vi "模拟量输入自动测试一组_fast_OK.vi"(8 "AD选择？":bool, 9 "DSP选择？":bool, 11 "第几个":i32) -> ()   [LabVIEW 2010]
panel:
  in  "AD测试值":dbl[](array[numeric])
  in  "DSP测试值":dbl[](array[numeric])
  # "从0开始"
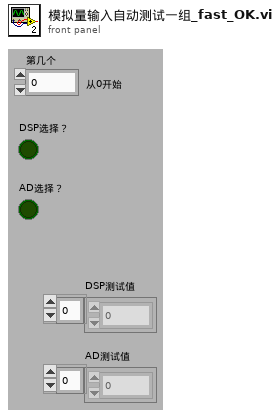
[diagram p1: front panel]
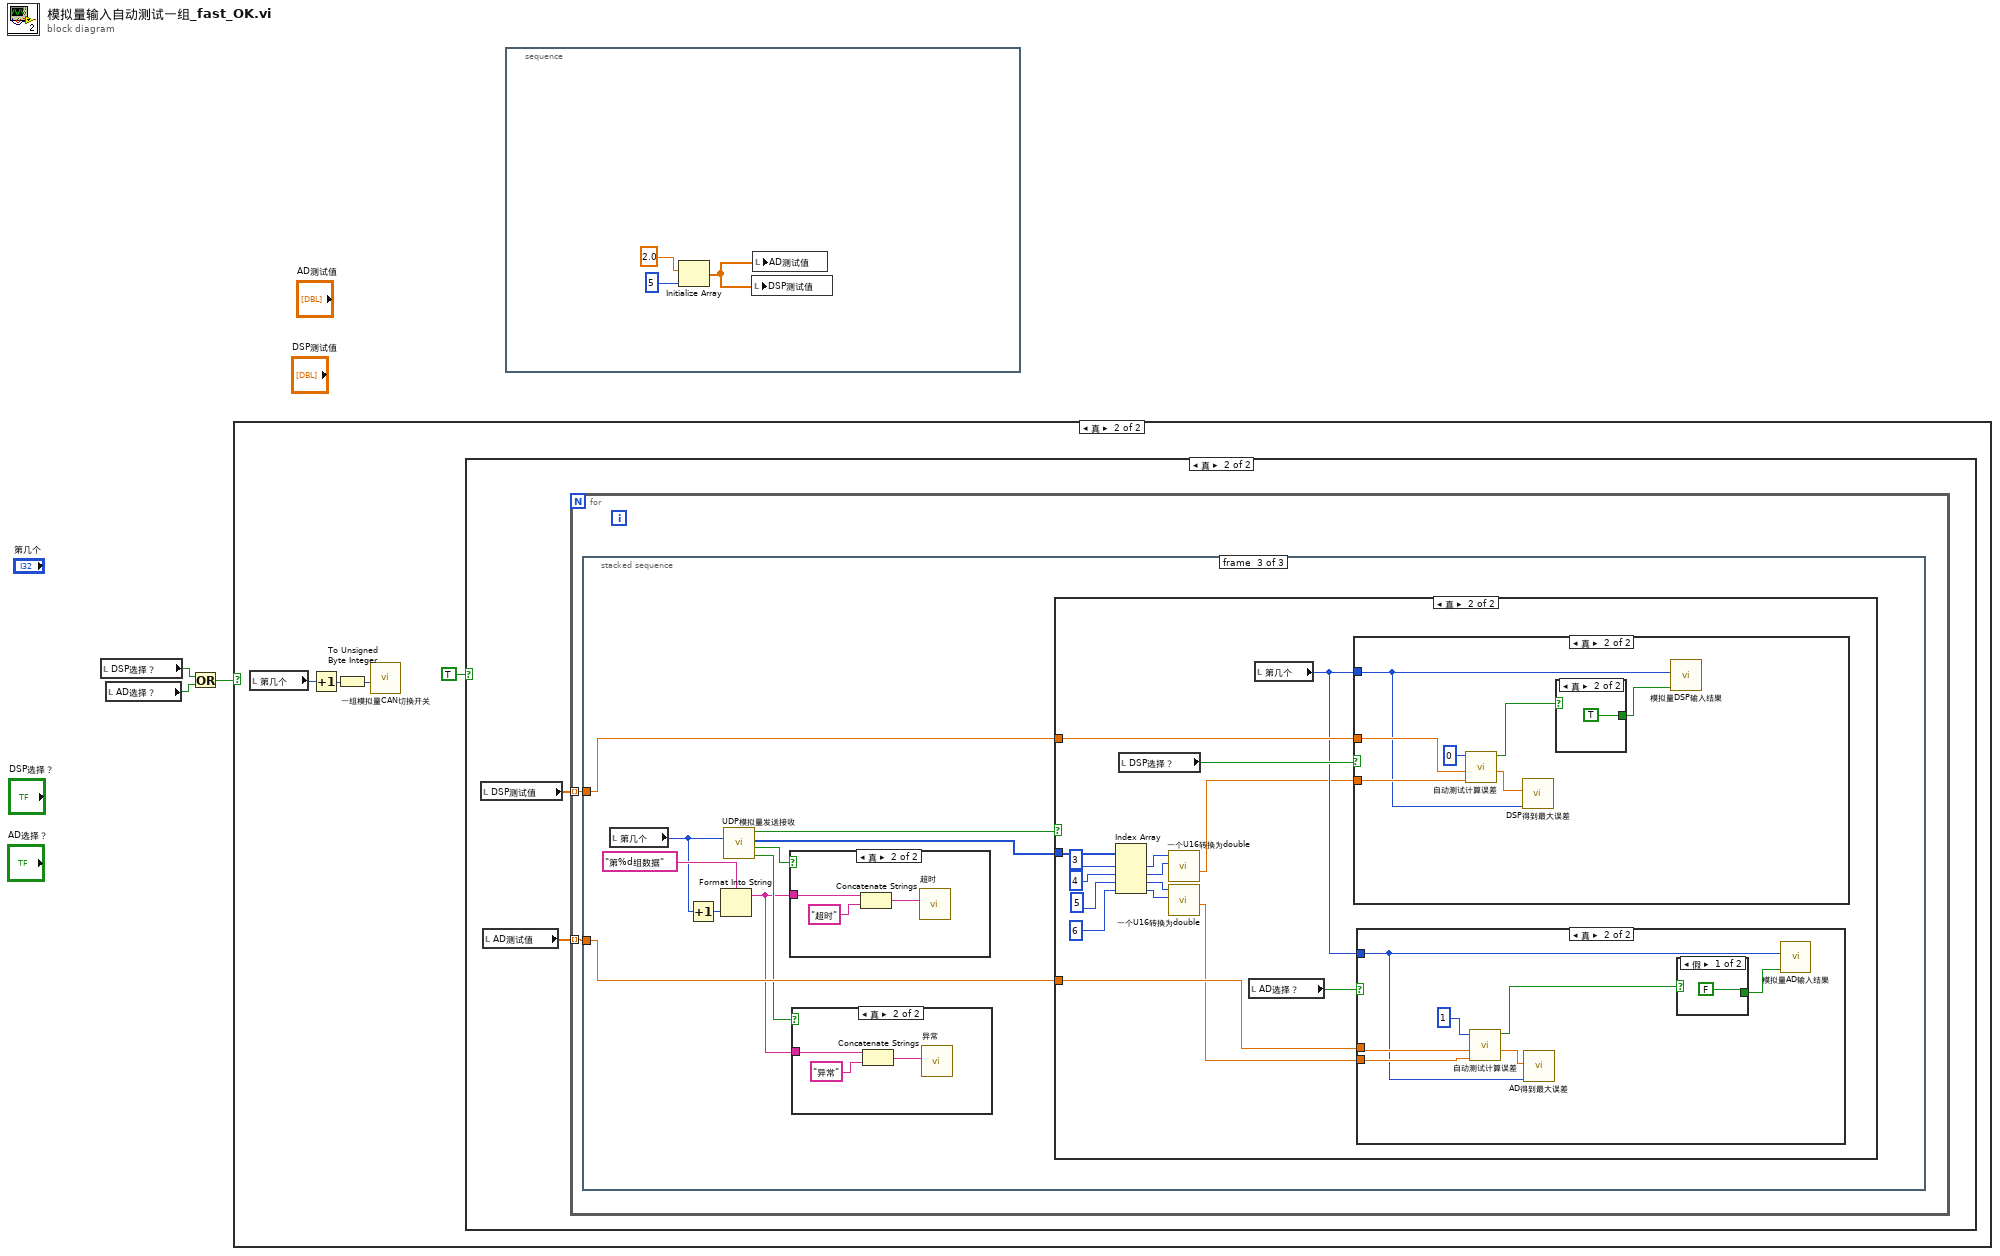
[diagram p0: block diagram]
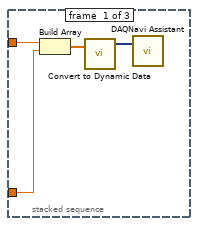
[diagram p4: hidden frame]
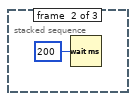
[diagram p5: hidden frame]
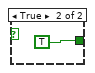
[diagram p10: hidden frame]
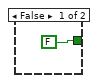
[diagram p12: hidden frame]
diagram:
  n1 = local read "DSP选择？"() -> (w2:bool)
  n2 = local read "AD选择？"() -> (w3:bool)
  n3 = Or(x=w2, y=w3) -> (x .or. y?=w1:bool)
  n4 = case shown="真" w1 {
    frame False {
    }
    frame True {
      n5 = local read "第几个"() -> (w7:i32)
      n6 = Increment(x=w7) -> (x+1=w5:i32)
      n7 = To Unsigned Byte Integer(number=w5) -> (unsigned 8bit integer=w6:u8)
      n8 = call "一组模拟量CAN切换开关.vi"("第几组数据"=w6) -> ()  [unwired: 10 in, 1 out]
      n9 = case shown="真" TRUE {
        frame False {
        }
        frame True {
          n10 = local read "DSP测试值"() -> (w9:dbl[])
          n11 = local read "AD测试值"() -> (w8:dbl[])
          n12 = for {
            tunnel: w9 -> [w11] mode=indexing
            tunnel: w8 -> [w10] mode=indexing
            n13 = stacked-sequence {
              tunnel: w11 -> [w13 _ w26]
              tunnel: w10 -> [w12 _ w25]
              frame #0 {
                n14 = Build Array(w13, w12) -> (w15:dbl[])
                n15 = call "Convert to Dynamic Data"("Array"=w15) -> ("Dynamic Data Type"=w14:dynamicdata)  [unwired: 3 out]
                n16 = call "DAQNavi Assistant"("data in(DDT)"=w14) -> ()  [unwired: 2 in, 17 out]
              }
              frame #1 {
                n17 = Wait (ms)(milliseconds to wait=u32 200 ("等待时间（毫秒）")) -> ()  [unwired: 1 out]
              }
              frame #2 {
                n18 = local read "第几个"() -> (w17:i32)
                n19 = Increment(x=w17) -> (x+1=w18:i32)
                n20 = Format Into String(format string="第%d组数据" ("格式字符串"), w18) -> (resulting string=w19:string)  [unwired: 2 in, 1 out]
                n21 = call "UDP模拟量发送接收.vi"("第几组"=w17) -> ("异常_找到?"=w20:bool, "接收超时?"=w22:bool, "接收的一帧数据"=w24:u16[], "正常_找到?"=w23:bool)  [unwired: 7 in]
                n22 = case shown="真" w22 {
                  tunnel: w19 -> [_ w32]
                  frame False {
                  }
                  frame True {
                    n23 = Concatenate Strings(w32, "超时" ("格式字符串")) -> (w30:string)
                    n24 = call "超时"("Message"=w30) -> ()  [unwired: 9 in, 2 out]
                  }
                }
                n25 = case shown="真" w20 {
                  tunnel: w19 -> [_ w29]
                  frame False {
                  }
                  frame True {
                    n26 = Concatenate Strings(w29, "异常" ("格式字符串")) -> (w27:string)
                    n27 = call "异常"("Message"=w27) -> ()  [unwired: 9 in, 2 out]
                  }
                }
                n28 = case shown="真" w23 {
                  tunnel: w24 -> [_ w40]
                  tunnel: w26 -> [_ w38]
                  tunnel: w25 -> [_ w37]
                  frame False {
                  }
                  frame True {
                    n29 = Index Array(array=w40, index #1=3 ("索引"), index #2=4 ("索引"), index #3=5 ("索引"), index #4=6 ("索引")) -> (element #1=w45:u16, element #2=w46:u16, element #3=w47:u16, element #4=w48:u16)
                    n30 = local read "DSP选择？"() -> (w39:bool)
                    n31 = call "一个U16转换为double.vi"("低16位_1"=w46, "高16位_1"=w45) -> ("反馈值"=w33:dbl)  [unwired: 9 in]
                    n32 = call "一个U16转换为double.vi"("低16位_1"=w48, "高16位_1"=w47) -> ("反馈值"=w36:dbl)  [unwired: 9 in]
                    n33 = local read "AD选择？"() -> (w35:bool)
                    n34 = local read "第几个"() -> (w34:i32)
                    n35 = case shown="真" w39 {
                      tunnel: w38 -> [_ w63]
                      tunnel: w33 -> [_ w62]
                      tunnel: w34 -> [_ w58]
                      frame False {
                      }
                      frame True {
                        n36 = call "自动测试计算误差.vi"("反馈值"=w62, "输入值"=w63, "DSP_OR_AD"=0) -> ("误差"=w59:dbl, "合格？"=w61:bool)  [unwired: 7 in]
                        n37 = call "DSP得到最大误差.vi"("第几组"=w58, "新误差值"=w59) -> ()  [unwired: 10 in]
                        n38 = case shown="真" w61 {
                          tunnel: [FALSE TRUE] -> w60
                          frame False {
                          }
                          frame True {
                          }
                        }
                        n39 = call "模拟量DSP输入结果.vi"("合格?"=w60, "第几个"=w58) -> ()  [unwired: 10 in]
                      }
                    }
                    n40 = case shown="真" w35 {
                      tunnel: w37 -> [_ w53]
                      tunnel: w36 -> [_ w52]
                      tunnel: w34 -> [_ w49]
                      frame False {
                      }
                      frame True {
                        n41 = call "自动测试计算误差.vi"("反馈值"=w52, "输入值"=w53, "DSP_OR_AD"=1) -> ("误差"=w50:dbl, "合格？"=w54:bool)  [unwired: 7 in]
                        n42 = call "AD得到最大误差.vi"("第几组"=w49, "新误差值"=w50) -> ()  [unwired: 10 in]
                        n43 = case shown="假" w54 {
                          tunnel: [FALSE TRUE] -> w51
                          frame False {
                          }
                          frame True {
                          }
                        }
                        n44 = call "模拟量AD输入结果.vi"("合格?"=w51, "第几个"=w49) -> ()  [unwired: 10 in]
                      }
                    }
                  }
                }
              }
            }
          }
        }
      }
    }
  }
  n45 = stacked-sequence {
    frame #0 {
      n46 = Initialize Array(2.0, 5 ("维数大小")) -> (w67:dbl[])
      n47 = local write "DSP测试值"(w67) -> ()
      n48 = local write "AD测试值"(w67) -> ()
    }
  }
